vi "InitCVT.vi"(8 "error in":errorcluster, 11 "DoNotSetChannels[]":string[](array[string])) -> (0 "error out":errorcluster)   [LabVIEW 2013, in "Picomotor8752.lvclass"]
uses:
  Picomotor8752.lvclass
  shared/CompressAndUpdate(Poly)/CompressAndUpdate(Numeric).vi
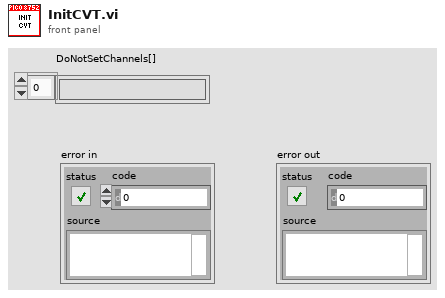
[diagram p1: front panel]
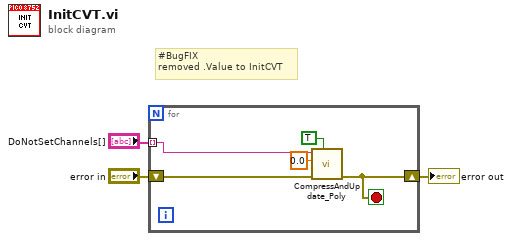
[diagram p0: block diagram]
diagram:
  # "#BugFIX\nremoved .Value to InitCVT"
  n1 = for {
    tunnel: "DoNotSetChannels[]" -> [w4] mode=indexing
    shift-right: [w6] -> w2
    shift-left: "error in" -> [w5]
    stop <- w6 stop-if-true
    n2 = call-poly "CompressAndUpdate_Poly.vi"("force CVT update (false)"=TRUE, "error in"=w5, "Numeric"=0.0, "command or variable name"=w4) -> ("error out"=w6:errorcluster)  [unwired: 7 in]
  }
  "error out" <- w2
